vi "Open Dialog VI.vi"(8 "error in":errorcluster, 9 "Windows title":string, 10 "ref for signalling":refnum<vi>, 11 "vi path":path=path "Display Settings.vi") -> (0 "error out":errorcluster)   [LabVIEW 2014, in "POLARIS Vision utility.lvlib"]
uses:
  POLARIS Vision utility.lvlib
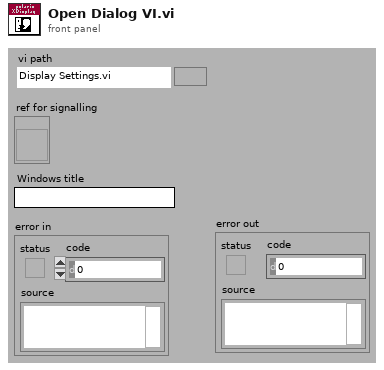
[diagram p1: front panel]
types:
  T1 = enum32{"Invalid", "Standard", "Closed", "Hidden", "Minimized", "Maximized"}
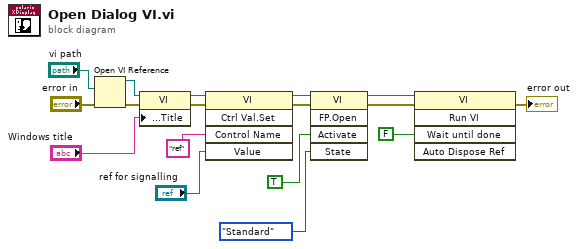
[diagram p0: block diagram]
diagram:
  n1 = Open VI Reference(vi path="vi path", error in (no error)="error in") -> (vi reference=w12:refnum<vi>, error out=w13:errorcluster)  [unwired: 4 in]
  n2 = property class="VI"(reference=w12, error in=w13, "Front Panel.Title"="Windows title") -> (reference out=w3:refnum<vi>, error out=w15:errorcluster)
  n3 = invoke class="VI" method="Ctrl Val.Set"(reference=w3, error in=w15, "Control Name"="ref", "Value"="ref for signalling") -> (reference out=w16:refnum<vi>, error out=w17:errorcluster)  [unwired: 1 in, 3 out]
  n4 = invoke class="VI" method="FP.Open"(reference=w16, error in=w17, "Activate"=TRUE ("Activate?"), "State"=T1."Standard") -> (reference out=w8:refnum<vi>, error out=w9:errorcluster)  [unwired: 1 in, 3 out]
  n5 = invoke class="VI" method="Run VI"(reference=w8, error in=w9, "Wait until done"=FALSE ("Wait Until Done")) -> (error out=→"error out":errorcluster)  [unwired: 2 in, 4 out]
